vi "Broadcast Batch Messages.vi"(8 "error in (no error)":errorcluster, 10 "Messages In":refnum<class "Message.lvclass">[](array[class]), 11 "Map Tree Queue Messenger in":refnum<class "Map Tree Queue Messenger.lvclass">) -> (0 "error out":errorcluster, 3 "Map Tree Queue Messenger out":refnum<class "Map Tree Queue Messenger.lvclass">)   [LabVIEW 2019, in "Map Tree Queue Messenger.lvclass"]
uses:
  Map Tree Queue Messenger.lvclass
  C:/Users/User/Desktop/Bussiness/Multi SPIM/General Library/Ancestor Class/Messenger/Messenger Map Composite/Messenger Map Composite.lvclass
  Ancestor Class/Message/Message.lvclass
  Map Tree Queue Messenger.lvclass/Map Tree Queue Messenger.ctl
  Ancestor Class/Messenger/Messenger Map Composite/Messenger Map Composite.lvclass/Messenger Map Composite.ctl
  Ancestor Class/Messenger/Messenger Map Composite/Public Data/Read Child Nodes.vi
  Ancestor Class/Messenger/Messenger/Messenger.lvclass
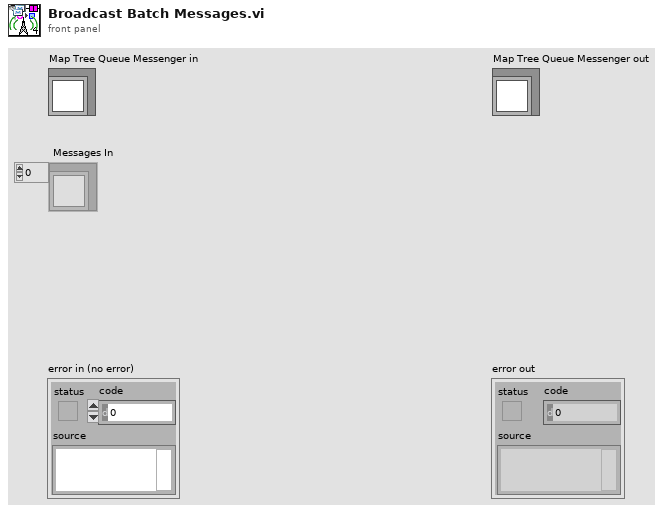
[diagram p1: front panel]
types:
  T1 = typedef "Message Queue.ctl" = refnum<queue>
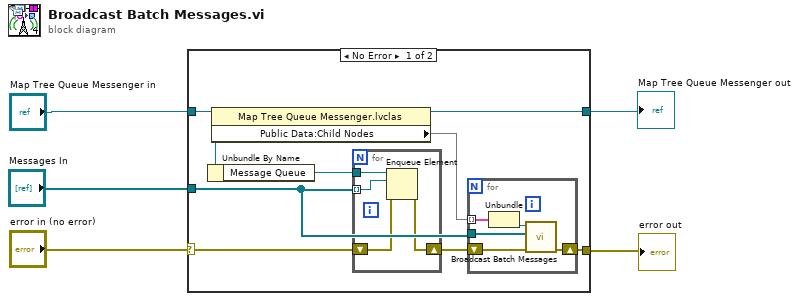
[diagram p0: block diagram]
diagram:
  n1 = case shown="No Error" "error in (no error)" {
    selector: "error in (no error)" -> [w12 w24]
    tunnel: [w10 w24] -> w2
    tunnel: [w6 w23] -> w4
    tunnel: "Map Tree Queue Messenger in" -> [w8 w23]
    tunnel: "Messages In" -> [w9 _]
    frame No Error {
      n2 = Unbundle By Name(w8) -> ("Message Queue"=w13:T1)
      n3 = property class="Map Tree Queue Messenger.lvclas"(reference=w8) -> (reference out=w6:refnum<class "Map Tree Queue Messenger.lvclass">, "Public Data:Child Nodes"=w7:map{i64, refnum<class "Messenger.lvclass">})  [unwired: 1 in, 1 out]
      n4 = for {
        tunnel: w13 -> [w22]
        tunnel: w9 -> [w21] mode=indexing
        shift-right: [w19] -> w11
        shift-left: w12 -> [w20]
        n5 = Enqueue Element(queue=w22, element=w21, error in (no error)=w20) -> (error out=w19:errorcluster)  [unwired: 1 in, 2 out]
      }
      n6 = for {
        shift-right: [w16] -> w10
        shift-left: w11 -> [w17]
        tunnel: w7 -> [w15] mode=indexing
        tunnel: w9 -> [w18]
        n7 = Unbundle(w15) -> ("Messenger"=w14:refnum<class "Messenger.lvclass">)  [unwired: 1 out]
        n8 = call-dynamic "Broadcast Batch Messages.vi"("error in (no error)"=w17, "Messages In"=w18, "Messenger in"=w14) -> ("error out"=w16:errorcluster)  [unwired: 7 in, 1 out]
      }
    }
    frame Error {
    }
  }
  "error out" <- w2
  "Map Tree Queue Messenger out" <- w4
